vi "PicoScope2000aAWG.vi"(6 "Arbitrary Waveform Settings":T2 {"Index Mode" items=["Single", "Dual", "Quad"]}, 7 "Standard Waveform Settings":T3={"Start Frequency"=1000.0, "Stop Frequency"=1000.0, "Increment"=0.0, "Dwell Time (seconds)"=0.0} {"Stop Frequency" min=0.03 max=1000000.0; "Start Frequency" min=0.03 max=1000000.0}, 8 "error in":errorcluster, 9 "General AWG Settings":T4={"Peak-to-Peak Voltage (microvolts)"=1000000, "Offset Voltage (microvolts)"=0, "Wave Type"=0, "Sweep Type"=0, "Shots"=0, "Sweeps"=0, "Trigger Type"=0, "Trigger Source"=0, "Ext. Threshold (ADC count)"=0, "White Noise"=FALSE} {"Trigger Source" items=["None", "Scope Trigger", "Aux. In", "Ext. In", "Software Trigger"]; "Trigger Type" items=["Rising", "Falling", "Gate High", "Gate Low"]; "Sweep Type" items=["Up", "Down", "Up-Down", "Down-Up"]; "Wave Type" items=["Sine"=0, "Square"=1, "Triangle"=2, "Ramp Up"=3, "Ramp Down"=4, "DC"=8, "Arbitrary"=6]}, 10 "Device Info":T1, 11 "Handle In":i16) -> (0 "error out":errorcluster, 1 "triggerSource":i32, 3 "Handle Out":i16, 4 "Arbitrary\nWaveform Graph":i16[](graph))   [LabVIEW 2010]
doc: "This VI can be used to control the arbitrary waveform generator. Standard waveforms can be selected or arbitrary waveform can be selected under 'Wave Type'. There are three settings clusters: general settings that apply to both arbitrary and standard waveforms, settings that apply only to standard waveforms and settings that apply only to arbitrary waveforms. It is not necessary to connect all of these clusters if only using arbitrary waveforms or only using standard waveforms are required.\n\nWhen selecting arbitrary waveform, it is necessary to specify a text file containing the wave form. This text file should have a single value on each line in the range -1 to 1. For further information on the settings, see descriptions of ps2000aSetSigGenBuiltIn and ps2000aSetSigGenArbitrary. SWG files from PicoScope software can loaded into this vi."
uses:
  ps2000a.dll
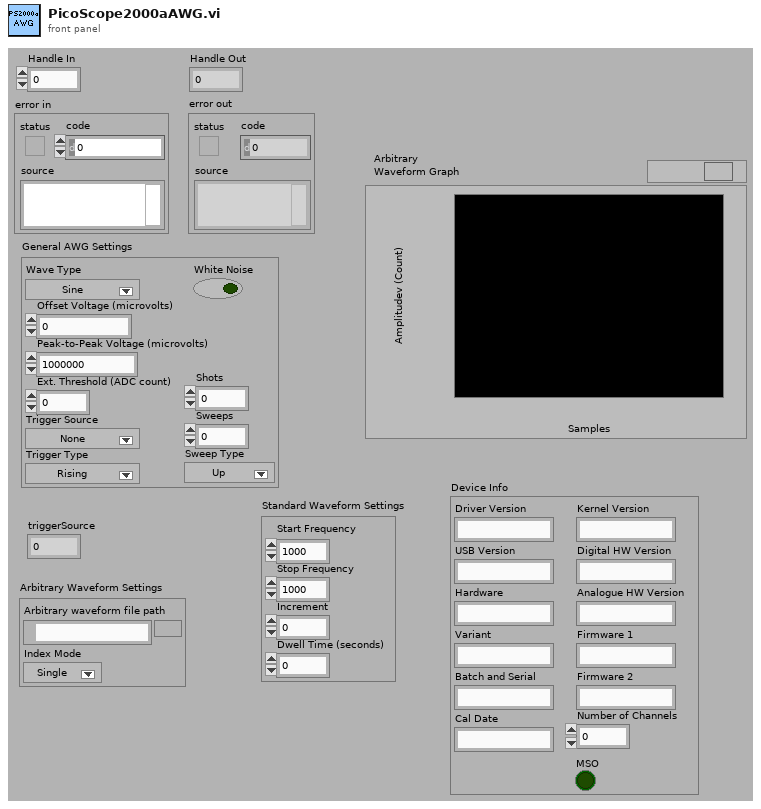
[diagram p1: front panel]
types:
  T1 = cluster{"Driver Version":string, "USB Version":string, "Hardware":string, "Variant":string, "Batch and Serial":string, "Cal Date":string, "Kernel Version":string, "Digital HW Version":string, "Analogue HW Version":string, "Firmware 1":string, "Firmware 2":string, "MSO":bool, "Number of Channels":i16}
  T2 = cluster{"Arbirary waveform file path":path, "Index Mode":u32}
  T3 = cluster{"Start Frequency":dbl, "Stop Frequency":dbl, "Increment":dbl, "Dwell Time (seconds)":dbl}
  T4 = cluster{"Peak-to-Peak Voltage (microvolts)":u32, "Offset Voltage (microvolts)":i32, "Wave Type":i16, "Sweep Type":i32, "Shots":u32, "Sweeps":u32, "Trigger Type":i32, "Trigger Source":i32, "Ext. Threshold (ADC count)":i16, "White Noise":bool}
  T5 = cluster{"status":bool, "code":u32, "source":string}
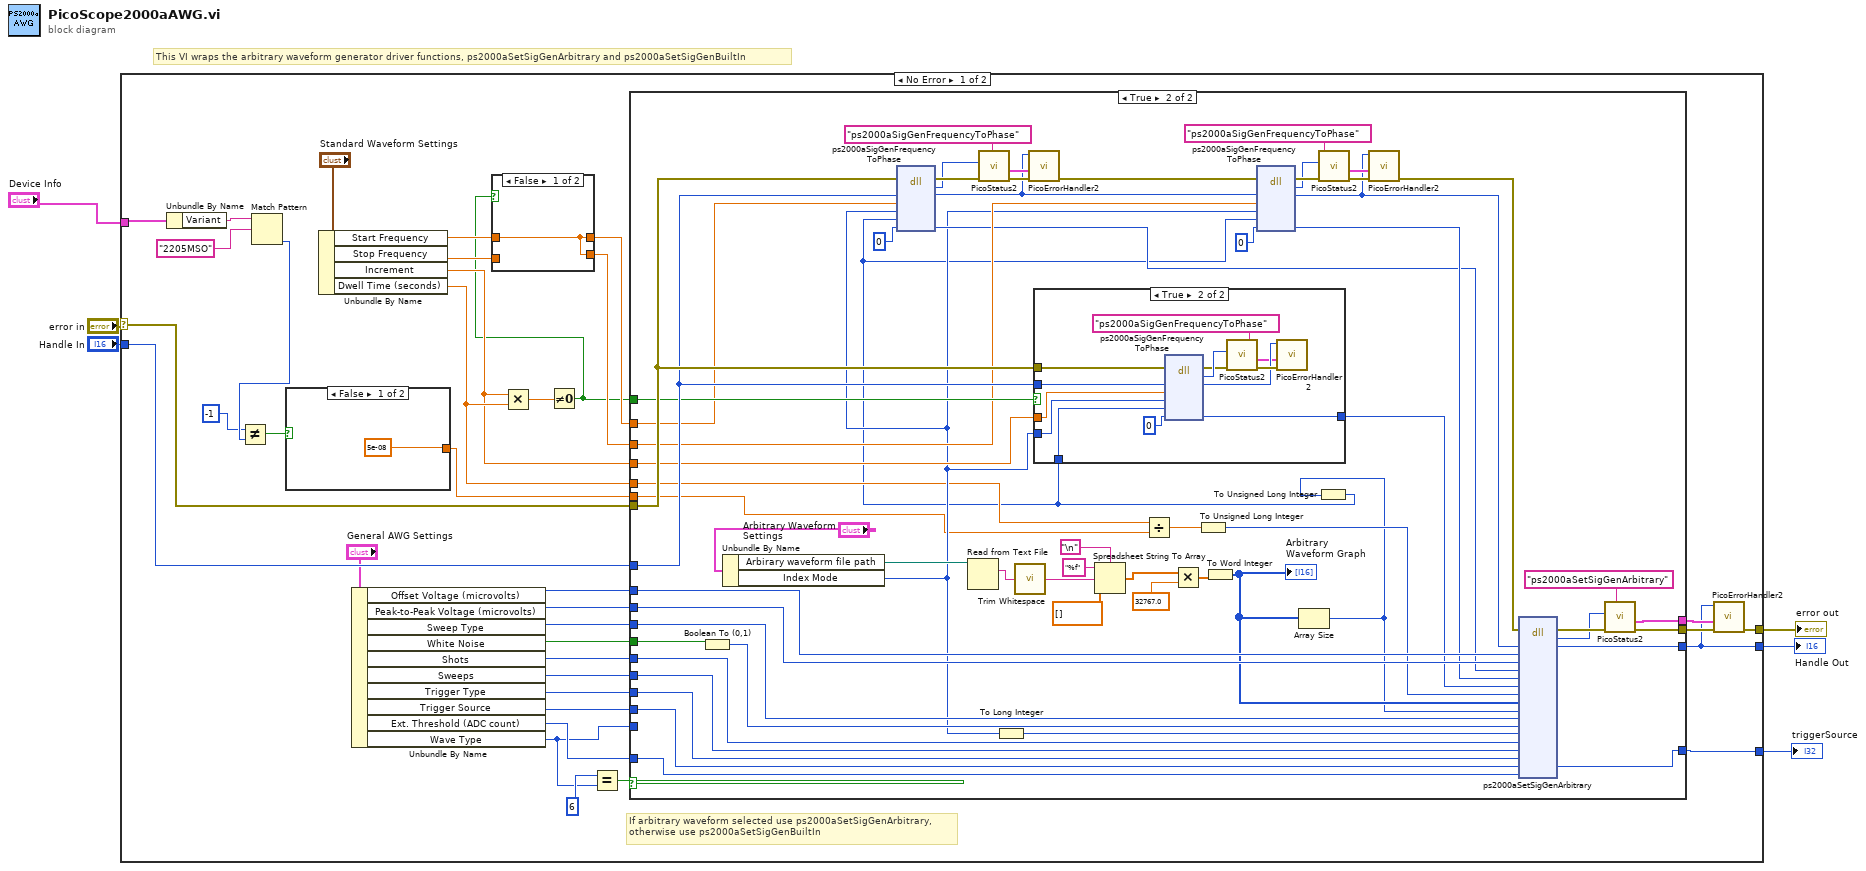
[diagram p0: block diagram]
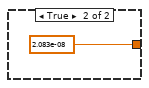
[diagram p2: hidden frame]
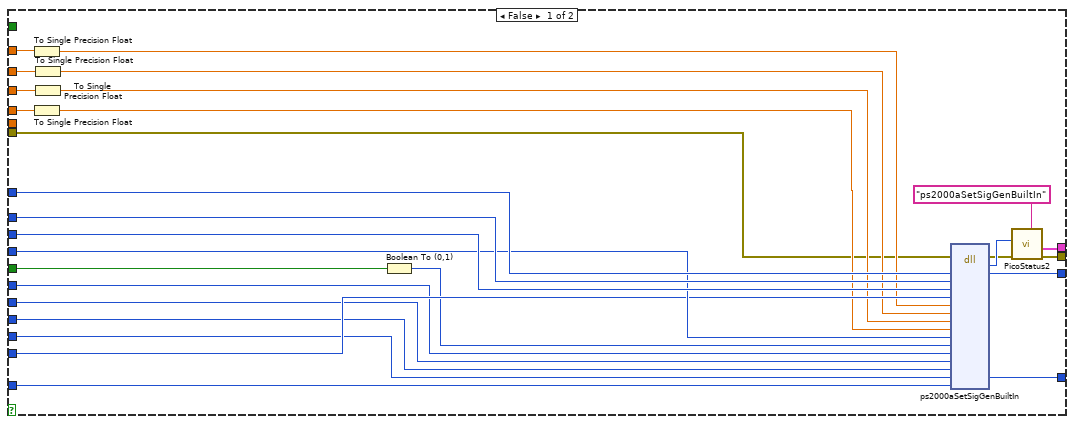
[diagram p4: hidden frame]
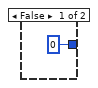
[diagram p5: hidden frame]
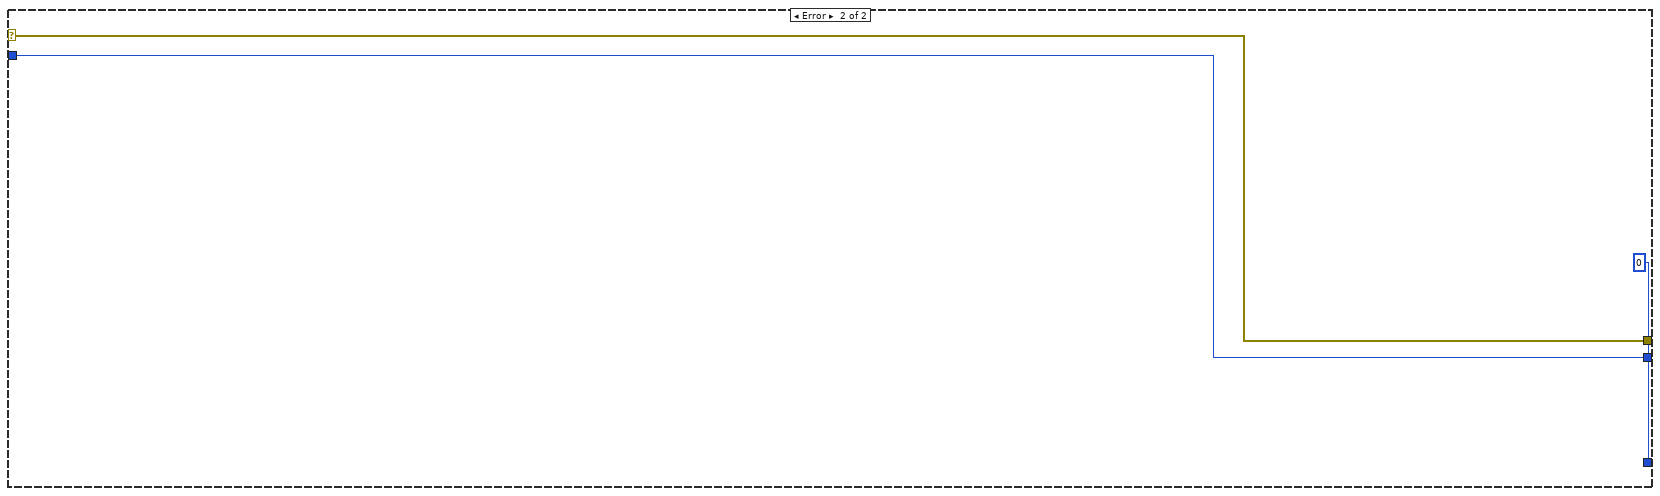
[diagram p6: hidden frame]
diagram:
  # "This VI wraps the arbitrary waveform generator driver functions, ps2000aSetSigGenArbitrary and ps2000aSetSigGenBuiltIn"
  n1 = case shown="No Error" "error in" {
    selector: "error in" -> [w22 w153]
    tunnel: [w7 w152] -> w6
    tunnel: "Handle In" -> [w40 w152]
    tunnel: [w38 w153] -> w4
    tunnel: [w26 0 ("triggerSource")] -> w2
    tunnel: "Device Info" -> [w11 _]
    frame No Error {
      # "If arbitrary waveform selected use ps2000aSetSigGenArbitrary, \notherwise use ps2000aSetSigGenBuiltIn"
      n2 = Unbundle By Name(w11) -> ("Variant"=w12:string)
      n3 = Match Pattern(string=w12, regular expression="2205MSO") -> (offset past match=w15:i32)  [unwired: 1 in, 3 out]
      n4 = Not Equal?(x=-1, y=w15) -> (x != y?=w10:bool)
      n5 = case shown="False" w10 {
        tunnel: [5e-08 ("y") 2.083e-08 ("y")] -> w9
        frame False {
        }
        frame True {
        }
      }
      n6 = Unbundle By Name("Standard Waveform Settings") -> ("Start Frequency"=w24:dbl, "Stop Frequency"=w23:dbl, "Increment"=w18:dbl, "Dwell Time (seconds)"=w19:dbl)
      n7 = Unbundle By Name("General AWG Settings") -> ("Offset Voltage (microvolts)"=w36:i32, "Peak-to-Peak Voltage (microvolts)"=w35:u32, "Sweep Type"=w34:i32, "White Noise"=w33:bool, "Shots"=w32:u32, "Sweeps"=w31:u32, "Trigger Type"=w30:i32, "Trigger Source"=w29:i32, "Ext. Threshold (ADC count)"=w28:i16, "Wave Type"=w27:i16)
      n8 = Multiply(x=w18, y=w19) -> (x*y=w17:dbl)
      n9 = Not Equal To 0?(x=w17) -> (x != 0?=w16:bool)
      n10 = case shown="False" w16 {
        tunnel: [w45 w47] -> w21
        tunnel: w23 -> [_ w47]
        tunnel: w24 -> [w45 w46]
        tunnel: [w45 w46] -> w20
        frame False {
        }
        frame True {
        }
      }
      n11 = Equal?(x=i16 6, y=w27) -> (x = y?=w42:bool)
      n12 = case shown="True" w42 {
        tunnel: [w75 w132] -> w7
        tunnel: w40 -> [w74 w101]
        tunnel: [w72 w130] -> w39
        tunnel: w36 -> [w70 w129]
        tunnel: w35 -> [w69 w128]
        tunnel: w34 -> [w68 w127]
        tunnel: w33 -> [w65 w126]
        tunnel: w32 -> [w64 w124]
        tunnel: w31 -> [w63 w123]
        tunnel: w30 -> [w62 w122]
        tunnel: w29 -> [w61 w121]
        tunnel: w28 -> [w60 w118]
        tunnel: w27 -> [w67 _]
        tunnel: [w59 w114] -> w26
        tunnel: w22 -> [w50 w102]
        tunnel: w19 -> [w58 w88]
        tunnel: w18 -> [w57 w97]
        tunnel: w21 -> [w56 w98]
        tunnel: w20 -> [w55 w99]
        tunnel: w16 -> [_ w100]
        tunnel: w9 -> [_ w87]
        tunnel: [w48 w80] -> w8
        frame False {
          n13 = To Single Precision Float(number=w55) -> (single precision float=w51:sgl)
          n14 = To Single Precision Float(number=w58) -> (single precision float=w54:sgl)
          n15 = To Single Precision Float(number=w56) -> (single precision float=w52:sgl)
          n16 = To Single Precision Float(number=w57) -> (single precision float=w53:sgl)
          n17 = Boolean To (0,1)(Boolean=w65) -> (0, 1=w66:i16)
          n18 = dll-call lib="ps2000a.dll" fn="ps2000aSetSigGenBuiltIn" ("ps3000.dll:_ps3000_open_unit@0")(error in=w50, "handle"=w74, "offsetVoltage"=w70, "pkToPk"=w69, "waveType"=w67, "startFrequency"=w51, "stopFrequency"=w52, "increment"=w53, "dwellTime"=w54, "sweepType"=w68, "whiteNoise"=w66, "shots"=w64, "sweeps"=w63, "triggerType"=w62, "triggerSource"=w61, "extInThreshold"=w60) -> (error out=w49:errorcluster, "PICO_STATUS"=w73:u32, "handle"=w75:i16, "triggerSource"=w59:i32)  [unwired: 15 in, 1 out]
          n19 = call "PicoStatus2.vi"("PICO source"="ps2000aSetSigGenBuiltIn" ("source"), "Error in"=w49, "PICO STATUS"=w73) -> ("error out"=w72:errorcluster, "PICO_STATUS out"=w48:T5)  [unwired: 5 in]
        }
        frame True {
          n20 = Boolean To (0,1)(Boolean=w126) -> (0, 1=w125:i16)
          n21 = Unbundle By Name("Arbitrary Waveform Settings") -> ("Arbirary waveform file path"=w119:path, "Index Mode"=w91:u32)
          n22 = Read from Text File(file (use dialog)=w119) -> (text=w86:string)  [unwired: 3 in, 3 out]
          n23 = To Long Integer(number=w91) -> (32bit integer=w90:i32)
          n24 = call <vilib>:"Trim Whitespace.vi"("string"=w86) -> ("trimmed string"=w85:string)  [unwired: 1 in]
          n25 = Spreadsheet String To Array(delimiter (Tab)="\n", format string="%f", spreadsheet string=w85, array type (2D Dbl)=dbl[] []) -> (array=w133:dbl[])
          n26 = Divide(x=w88, y=w87) -> (x/y=w79:dbl)
          n27 = Multiply(x=w133, y=32767.0 ("deltaPhaseIncrement")) -> (x*y=w115:dbl[])
          n28 = To Unsigned Long Integer(number=w79) -> (unsigned 32bit integer=w78:u32)
          n29 = To Word Integer(number=w115) -> (16bit integer=w117:i16[])
          "Arbitrary\nWaveform Graph" <- w117
          n30 = Array Size(array=w117) -> (size(s)=w76:i32)
          n31 = To Unsigned Long Integer(number=w76) -> (unsigned 32bit integer=w77:u32)
          n32 = dll-call lib="ps2000a.dll" fn="ps2000aSigGenFrequencyToPhase" ("ps3000.dll:_ps3000_open_unit@0")(error in=w102, "handle"=w101, "frequency"=w99, "indexMode"=w91, "bufferLength"=w77, "phase"=u32 0) -> (error out=w110:errorcluster, "PICO_STATUS"=w109:u32, "handle"=w82:i16, "phase"=w92:u32)  [unwired: 5 in, 1 out]
          n33 = call "PicoStatus2.vi"("PICO source"="ps2000aSigGenFrequencyToPhase" ("source"), "Error in"=w110, "PICO STATUS"=w109) -> ("error out"=w112:errorcluster, "PICO_STATUS out"=w84:T5)  [unwired: 5 in]
          n34 = call "PicoErrorHandler2.vi"("error in (no error)"=w112, "PICO_STATUS in"=w84, "handle In"=w82) -> ("error out"=w103:errorcluster)  [unwired: 8 in]
          n35 = case shown="True" w100 {
            tunnel: w102 -> [_ w146]
            tunnel: w101 -> [_ w145]
            tunnel: w97 -> [_ w144]
            tunnel: w77 -> [_ w142]
            tunnel: [u32 0 ("phase") w141] -> w93
            tunnel: w91 -> [_ w140]
            frame False {
            }
            frame True {
              n36 = dll-call lib="ps2000a.dll" fn="ps2000aSigGenFrequencyToPhase" ("ps3000.dll:_ps3000_open_unit@0")(error in=w146, "handle"=w145, "frequency"=w144, "indexMode"=w140, "bufferLength"=w142, "phase"=u32 0) -> (error out=w149:errorcluster, "PICO_STATUS"=w150:u32, "handle"=w139:i16, "phase"=w141:u32)  [unwired: 5 in, 1 out]
              n37 = call "PicoStatus2.vi"("PICO source"="ps2000aSigGenFrequencyToPhase" ("source"), "Error in"=w149, "PICO STATUS"=w150) -> ("error out"=w147:errorcluster, "PICO_STATUS out"=w138:T5)  [unwired: 5 in]
              n38 = call "PicoErrorHandler2.vi"("error in (no error)"=w147, "PICO_STATUS in"=w138, "handle In"=w139) -> ()  [unwired: 8 in, 1 out]
            }
          }
          n39 = dll-call lib="ps2000a.dll" fn="ps2000aSigGenFrequencyToPhase" ("ps3000.dll:_ps3000_open_unit@0")(error in=w103, "handle"=w82, "frequency"=w98, "indexMode"=w91, "bufferLength"=w77, "phase"=u32 0) -> (error out=w106:errorcluster, "PICO_STATUS"=w105:u32, "handle"=w81:i16, "phase"=w94:u32)  [unwired: 5 in, 1 out]
          n40 = call "PicoStatus2.vi"("PICO source"="ps2000aSigGenFrequencyToPhase" ("source"), "Error in"=w106, "PICO STATUS"=w105) -> ("error out"=w108:errorcluster, "PICO_STATUS out"=w83:T5)  [unwired: 5 in]
          n41 = call "PicoErrorHandler2.vi"("error in (no error)"=w108, "PICO_STATUS in"=w83, "handle In"=w81) -> ("error out"=w104:errorcluster)  [unwired: 8 in]
          n42 = dll-call lib="ps2000a.dll" fn="ps2000aSetSigGenArbitrary" ("ps3000.dll:_ps3000_open_unit@0")(error in=w104, "handle"=w81, "offsetVoltage"=w129, "pkToPk"=w128, "startDeltaPhase"=w92, "stopDeltaPhase"=w94, "deltaPhaseIncrement"=w93, "dwellCount"=w78, "arbitraryWaveform"=w117, "arbitraryWaveformSize"=w76, "sweepType"=w127, "whiteNoise"=w125, "indexMode"=w90, "shots"=w124, "sweeps"=w123, "triggerType"=w122, "triggerSource"=w121, "extInThreshold"=w118) -> (error out=w113:errorcluster, "PICO_STATUS"=w89:u32, "handle"=w132:i16, "triggerSource"=w114:i32)  [unwired: 17 in, 1 out]
          n43 = call "PicoStatus2.vi"("PICO source"="ps2000aSetSigGenArbitrary" ("source"), "Error in"=w113, "PICO STATUS"=w89) -> ("error out"=w130:errorcluster, "PICO_STATUS out"=w80:T5)  [unwired: 5 in]
        }
      }
      n44 = call "PicoErrorHandler2.vi"("error in (no error)"=w39, "PICO_STATUS in"=w8, "handle In"=w7) -> ("error out"=w38:errorcluster)  [unwired: 8 in]
    }
    frame Error {
    }
  }
  "Handle Out" <- w6
  "error out" <- w4
  "triggerSource" <- w2
